vi "节点转换.vi"(11 "节点":T2(array[cluster]) {"ID" format="%02x"}) -> (3 "节点-输出":T1(array[cluster]))   [LabVIEW 2019]
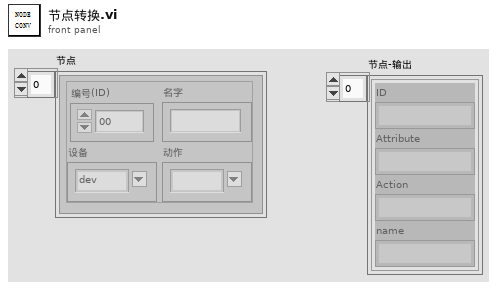
[diagram p1: front panel]
types:
  T1 = cluster{"ID":string, "Attribute":string, "Action":string, "name":string}[]
  T2 = cluster{"ID":u8, "Attribute":string, "Action":string, "name":string}[]
  T3 = cluster{"ID":string, "Attribute":string, "Action":string, "name":string}
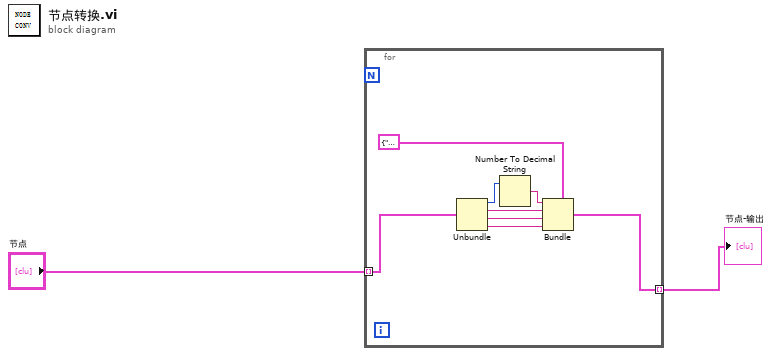
[diagram p0: block diagram]
diagram:
  n1 = for {
    tunnel: "节点" -> [w4] mode=indexing
    tunnel: [w3] -> w1 mode=indexing
    n2 = Unbundle(w4) -> ("ID"=w5:u8, "Attribute"=w7:string, "Action"=w8:string, "name"=w9:string)
    n3 = Number To Decimal String(number=w5) -> (decimal integer string=w6:string)  [unwired: 1 in]
    n4 = Bundle(cluster=T3 {"ID"="", "Attribute"="", "Action"="", "name"=""} ("node"), "ID"=w6, "Attribute"=w7, "Action"=w8, "name"=w9) -> (w3:T3)
  }
  "节点-输出" <- w1
